vi "Button.vi"(10 "Button":bool, 11 "Ex Event Actor in":refnum<class "Ex Event Actor.lvclass">) -> (0 "error out":errorcluster)   [LabVIEW 2021, in "Ex Event Actor.lvlib" / "Ex Event Actor.lvclass"]
uses:
  Ex Event Actor.lvclass
  Ex Event Actor.lvclass/Ex Event Actor.ctl
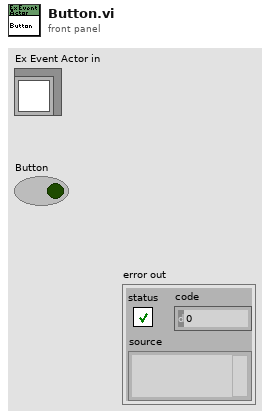
[diagram p1: front panel]
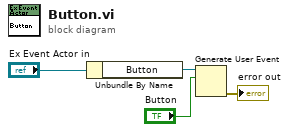
[diagram p0: block diagram]
diagram:
  n1 = Unbundle By Name("Ex Event Actor in") -> ("Button"=w3:refnum<user-event>)
  n2 = Generate User Event(user event=w3, event data cluster="Button") -> (error out=→"error out":errorcluster)  [unwired: 2 in, 1 out]
